vi "cRIOSystemInfo.vi"(8 "error in (no error)":errorcluster, 11 "session in":refnum<k21>="localhost") -> (0 "error out":errorcluster, 2 "system info":T1)   [LabVIEW 2017, in "cRIODetectHW.lvlib"]
doc: "Gets information about the controller, chassis, or modules."
uses:
  <vilib>/addons/cRIODetectHW/cRIODetectHW.lvlib
  <vilib>/addons/cRIODetectHW/control/SystemHW.ctl
  <vilib>/addons/cRIODetectHW/control/cRIO Product Info.ctl
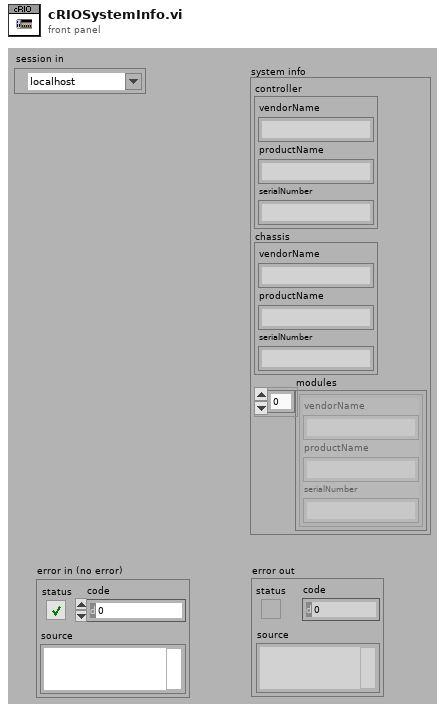
[diagram p1: front panel]
types:
  T1 = typedef "cRIODetectHW.lvlib/SystemHW.ctl" = cluster{"controller":T2, "chassis":T2, "modules":T2[]}
  T2 = typedef "cRIODetectHW.lvlib/cRIO Product Info.ctl" = cluster{"vendorName":string, "productName":string, "serialNumber":string}
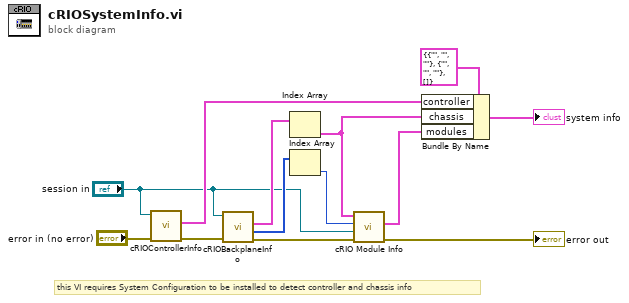
[diagram p0: block diagram]
diagram:
  # "this VI requires System Configuration to be installed to detect controller and chassis info"
  n1 = call <vilib>:"cRIOControllerInfo.vi"("error in (no error)"="error in (no error)", "session in"="session in") -> ("error out"=w13:errorcluster, "cRIO Controller Information"=w7:T2)  [unwired: 8 in]
  n2 = call <vilib>:"cRIOBackplaneInfo.vi"("error in (no error)"=w13, "session in"="session in") -> ("error out"=w10:errorcluster, "Number of Slots"=w3:i32[], "Chasses Info"=w12:T2[])  [unwired: 7 in]
  n3 = Index Array(array=w12) -> (element=w4:T2)  [unwired: 1 in]
  n4 = Index Array(array=w3) -> (element=w2:i32)  [unwired: 1 in]
  n5 = call <vilib>:"cRIO Module Info.vi"("error in (no error)"=w10, "session"="session in", "number of slots"=w2, "cRIO Backplane"=w4) -> ("error out"=→"error out":errorcluster, "cRIO Modules"=w6:T2[])  [unwired: 6 in]
  n6 = Bundle By Name(cluster=T1 {"controller"={"vendorName"="", "productName"="", "serialNumber"=""}, "chassis"={"vendorName"="", "productName"="", "serialNumber"=""}, "modules"=[]} ("SystemHW"), "controller"=w7, "chassis"=w4, "modules"=w6) -> (→"system info":T1)
